vi "FPGA_Open.vi"(2 "error in":errorcluster) -> (0 "error out":errorcluster)   [LabVIEW 2009, in "FPGA.lvlib"]
uses:
  FPGA.lvlib
  <vilib>/rvi/interface/nirviOpenFPGA/nirviOpenFPGA.xnode
  FPGA Bitfiles/scmproject.lvproj_FPGA Target_RobotFPGA.vi.lvbitx
  RobotFPGA.vi
  <vilib>/FPGAPlugInAG/cRIO-9074/nirviIntfOpen_cRIO-9074.vi
  <vilib>/userDefined/High Color/nirio_resource_hc.ctl
  Utility.lvlib
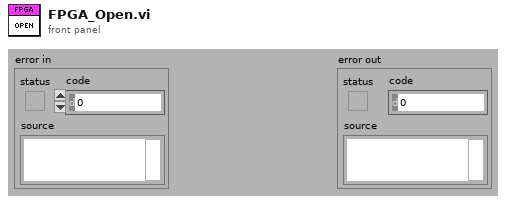
[diagram p1: front panel]
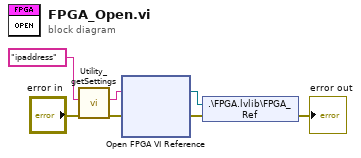
[diagram p0: block diagram]
diagram:
  n1 = call "Utility_getSettings.vi"("error in"="error in", "Search Setting String"="ipaddress") -> ("errorout"=w3:errorcluster, "Setting Value"=w2:string)  [unwired: 7 in, 1 out]
  n2 = xnode "Open FPGA VI Reference"("error in"=w3, "resource name"=w2) -> ("FPGA VI Reference Out"=w7:refnum<k20>, "error out"=w6:errorcluster)
  n3 = shared-variable ".\\FPGA.lvlib\\FPGA_Ref"(w7, error in=w6) -> (error out=→"error out":errorcluster)
